vi "WaitUntilDone.vi"(8 "error in (no error)":errorcluster, 10 "control register address":u32, 11 "sessionID in":u32) -> (0 "error out":errorcluster, 3 "sessionID out":u32)   [LabVIEW 2020, in "NI_TargetHelper.lvlib"]
uses:
  <vilib>/TargetSupport/NI_TargetHelper/NI_TargetHelper.lvlib
  NiFpgaLv.dll
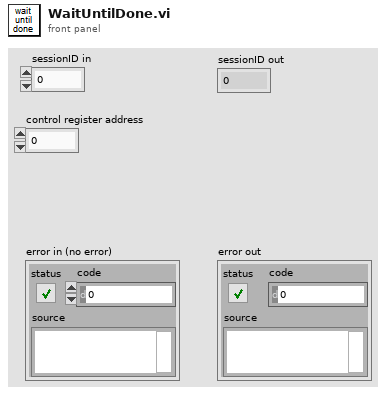
[diagram p1: front panel]
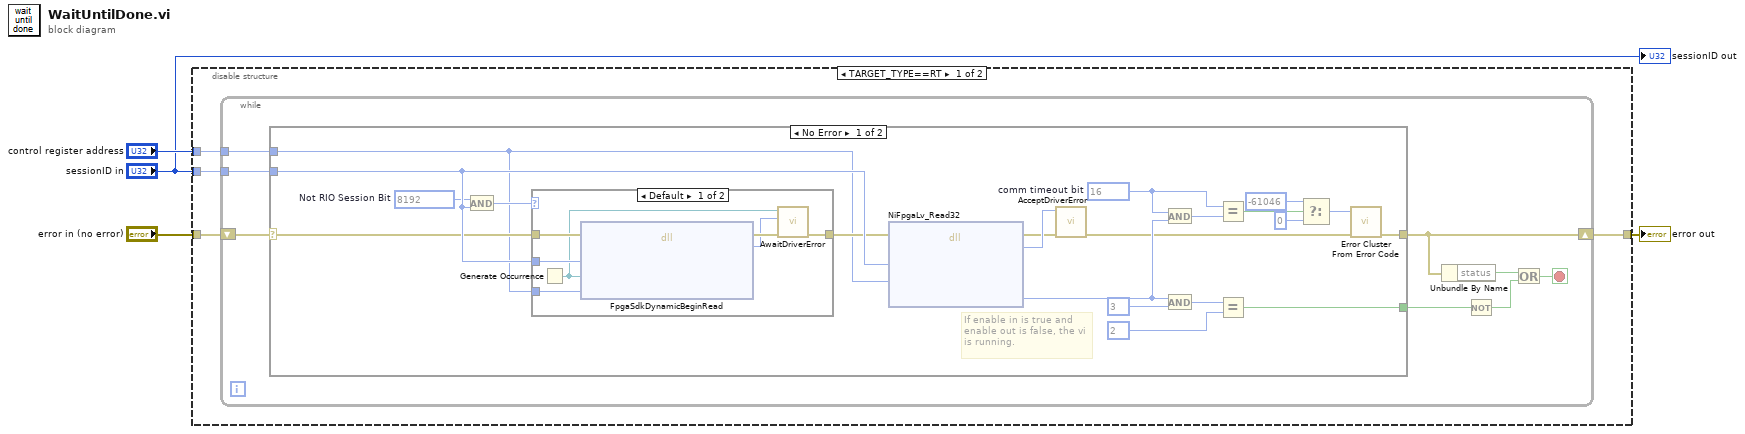
[diagram p0: block diagram]
diagram:
  n1 = disable-structure shown="TARGET_TYPE==RT" {
    disable-tunnel: "error in (no error)" -> [w8 _]
    disable-tunnel: "control register address" -> [w7 _]
    disable-tunnel: [w6 _] -> w2
    disable-tunnel: "sessionID in" -> [w5 _]
    frame condition #0 {
      n2 = while {
        tunnel: w5 -> [w9]
        shift-right: [w12] -> w6
        shift-left: w8 -> [w13]
        tunnel: w7 -> [w11]
        stop <- w14 stop-if-true
        n3 = case shown="No Error" w13 {
          selector: w13 -> [w27 w46]
          tunnel: w9 -> [w28 _]
          tunnel: [w32 w46] -> w12
          tunnel: w11 -> [w17 _]
          tunnel: [w25 _] -> w10
          frame No Error {
            w22 = u32 8192  # Not RIO Session Bit
            w36 = u32 16  # comm timeout bit
            # "If enable in is true and\nenable out is false, the vi\nis running."
            n4 = And(x=w22, y=w28) -> (x .and. y?=w21:u32)
            n5 = case shown="Default" w21 {
              tunnel: w27 -> [w44 w45]
              tunnel: [w40 w45] -> w23
              tunnel: w28 -> [w43 _]
              tunnel: w17 -> [w42 _]
              frame Default {
                n6 = Generate Occurrence() -> (w39:refnum<k4>)
                n7 = dll-call lib="LabVIEW" fn="FpgaSdkDynamicBeginRead"(error in=w44, "session"=w43, "occurrence"=w39, "index"=w42) -> (error out=w41:errorcluster, "status"=w38:i32)  [unwired: 5 in, 1 out]
                n8 = call <vilib>:"AwaitDriverError.vi"("error in (no error)"=w41, "status"=w38, "Occurrence in"=w39) -> ("error out"=w40:errorcluster)  [unwired: 8 in]
              }
              frame 0 {
              }
            }
            n9 = dll-call lib="NiFpgaLv.*" fn="NiFpgaLv_Read32" label="niLvFpgaRead32"(error in=w23, "session"=w28, "address"=w17) -> (error out=w19:errorcluster, "status"=w20:i32, "value"=w26:u32)  [unwired: 5 in, 1 out]
            n10 = call <vilib>:"AcceptDriverError.vi"("error in (no error)"=w19, "status"=w20) -> ("error out"=w18:errorcluster)  [unwired: 9 in]
            n11 = And(x=w36, y=w26) -> (x .and. y?=w37:u32)
            n12 = And(x=w26, y=u32 3) -> (x .and. y?=w30:u32)
            n13 = Equal?(x=w36, y=w37) -> (x = y?=w24:bool)
            n14 = Equal?(x=w30, y=u32 2) -> (x = y?=w25:bool)
            n15 = Select(t=-61046 ("error code (0)"), s=w24, f=0 ("error code (0)")) -> (s? t:f=w33:i32)
            n16 = call <vilib>:"Error Cluster From Error Code.vi"("error in (no error)"=w18, "error code (0)"=w33) -> ("error out"=w32:errorcluster)  [unwired: 1 in, 6 out]
          }
          frame Error {
          }
        }
        n17 = Unbundle By Name(w12) -> ("status"=w16:bool)
        n18 = Not(x=w10) -> (.not. x?=w15:bool)
        n19 = Or(x=w16, y=w15) -> (x .or. y?=w14:bool)
      }
    }
    frame condition #1 (active) {
    }
  }
  "error out" <- w2
  "sessionID out" <- "sessionID in"
